vi "StateMachineTest.vi"() -> ()   [LabVIEW 2015]
uses:
  State Machine.lvlib
panel:
  in  "Initialize":bool
  in  "Stop":bool
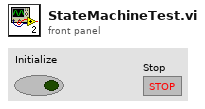
[diagram p1: front panel]
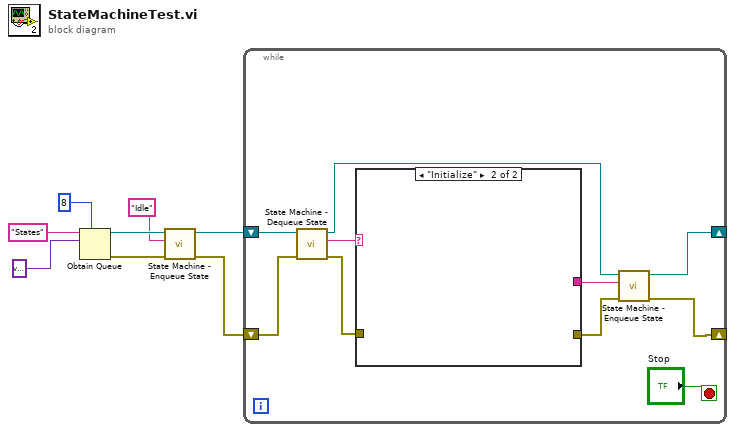
[diagram p0: block diagram]
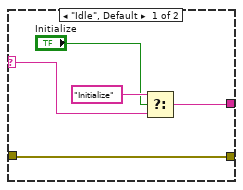
[diagram p2: hidden frame]
diagram:
  n1 = Obtain Queue(max queue size (-1, unlimited)=8, name (unnamed)="States", element data type=variant) -> (queue out=w5:refnum<queue>, error out=w4:errorcluster)  [unwired: 2 in, 1 out]
  n2 = call "State Machine - Enqueue State.vi"("error in (no error)"=w4, "State"="Idle", "Queue In"=w5) -> ("error out"=w1:errorcluster, "Queue Out"=w2:refnum<queue>)  [unwired: 7 in]
  n3 = while {
    shift-right: [w9] -> _
    shift-left: w2 -> [w17]
    shift-right: [w11] -> _
    shift-left: w1 -> [w16]
    stop <- "Stop" stop-if-true
    n4 = call "State Machine - Dequeue State.vi"("error in (no error)"=w16, "Queue In"=w17) -> ("error out"=w14:errorcluster, "State"=w18:string, "Queue Out"=w10:refnum<queue>)  [unwired: 5 in, 2 out]
    n5 = case shown="\"Initialize\"" w18 {
      selector: w18 -> [w22 _]
      tunnel: [w23 _] -> w12
      tunnel: w14 -> [w23 _]
      tunnel: [w19 _] -> w13
      frame "Idle", Default {
        n6 = Select(t="Initialize", s="Initialize", f=w22) -> (s? t:f=w19:string)
      }
      frame "Initialize" {
      }
    }
    n7 = call "State Machine - Enqueue State.vi"("error in (no error)"=w12, "State"=w13, "Queue In"=w10) -> ("error out"=w11:errorcluster, "Queue Out"=w9:refnum<queue>)  [unwired: 7 in]
  }
